vi "Build.vi"(6 "Version":T2, 7 "Build Events":refnum<class "Build Events API.lvclass">, 8 "error in (no error)":errorcluster, 10 "Build Info":T1, 11 "App Build in":refnum<class "App Build.lvclass">) -> (0 "error out":errorcluster)   [LabVIEW 2020, in "Builder Tools.lvlib" / "App Build.lvclass"]
uses:
  App Build.lvclass
  Builder Core/Version.ctl
  Build Events API/Build Events API.lvclass
  Build Info.ctl
  App Build.lvclass/App Build.ctl
  <vilib>/AppBuilder/AB_API_Simple/NI_App_Builder_API.lvlib
  <vilib>/AppBuilder/AB_API/Build/NI_AB_API_Build.lvclass
  <vilib>/AppBuilder/AB_API/common/AB_API Build Object Selector.ctl
  Builder Tools.lvlib
  <vilib>/AppBuilder/AB_API_Simple/Set Build Specification Version (path).vi
  Builder Core/Builder Core.lvlib
panel:
  out "Progress":i32
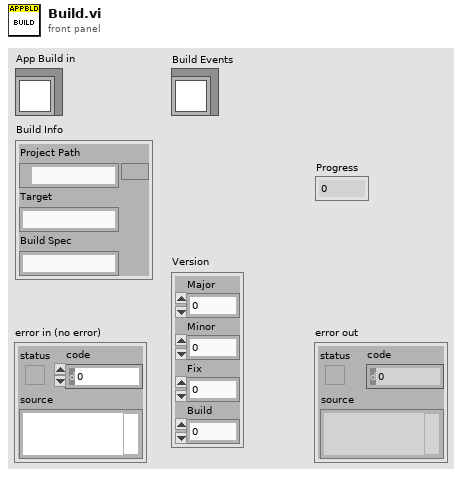
[diagram p1: front panel]
types:
  T1 = typedef "Builder Tools.lvlib/Build Info.ctl" = cluster{"Project Path":path, "Target":string, "Build Spec":string}
  T2 = typedef "Builder Core.lvlib/Version.ctl" = cluster{"Major":u16, "Minor":u16, "Fix":u16, "Build":u16}
  T3 = typedef "AB_API Build Object Selector.ctl" = enum16{"Source Distribution", "Deployable Source Distribution", "DLL", "EXE", "Packed Library", "Deployable Packed Library", "RT EXE", ".NET Interop Assembly"}
  T4 = typedef "AB_API ProgressBar_Events.ctl" = cluster{"newJob":refnum<user-event>, "newItem":refnum<user-event>, "errorMsg":T5, "cancel":refnum<user-event>}
  T5 = typedef "AB_API ProgressBar_BuildError.ctl" = refnum<user-event>
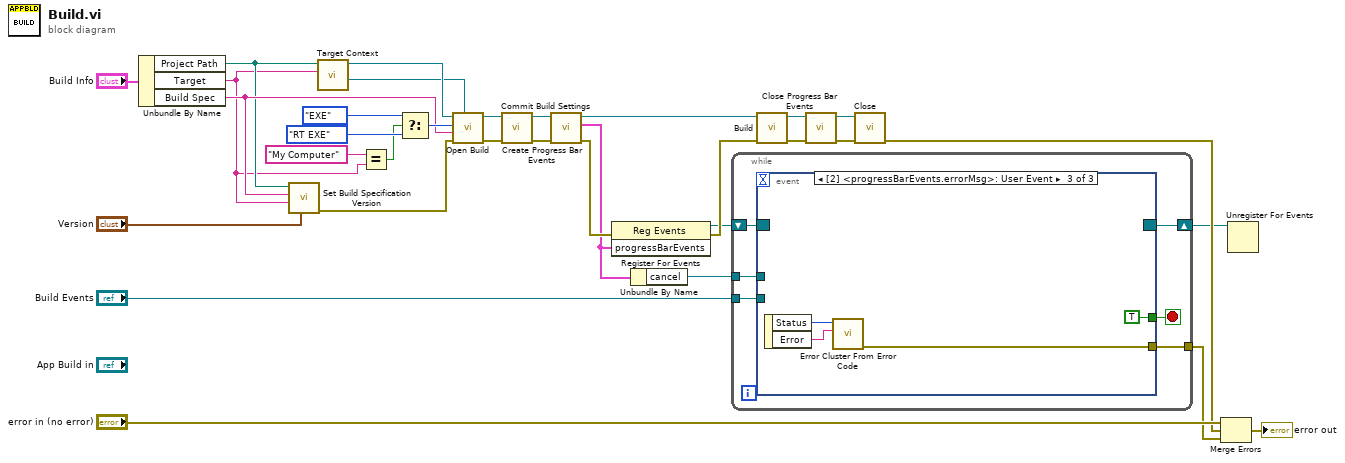
[diagram p0: block diagram]
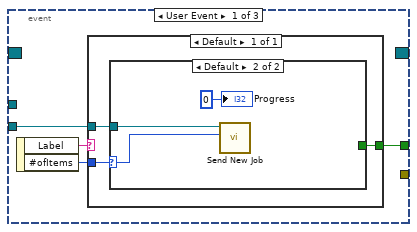
[diagram p2: hidden frame]
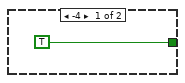
[diagram p3: hidden frame]
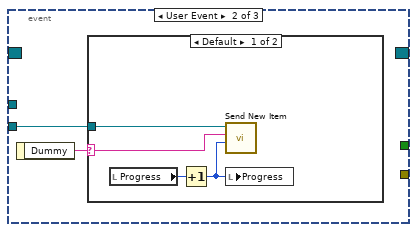
[diagram p4: hidden frame]
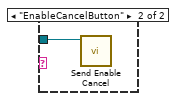
[diagram p5: hidden frame]
diagram:
  n1 = Unbundle By Name("Build Info") -> ("Project Path"=w22:path, "Target"=w21:string, "Build Spec"=w23:string)
  n2 = call-poly <vilib>:"Set Build Specification Version.vi"("Build Specification Version"="Version", "Name of target (My Computer)"=w21, "Name of build specification"=w23, "Path to project"=w22) -> ("error out"=w24:errorcluster)  [unwired: 7 in]
  n3 = call "Target Context.vi"("Target Name"=w21, "Project Path"=w22) -> ("Target"=w19:refnum<vi>, "Project"=w20:refnum<vi>)  [unwired: 7 in, 1 out]
  n4 = Equal?(x="My Computer", y=w21) -> (x = y?=w26:bool)
  n5 = Select(t=AB_API_Build_Object_Selector."EXE" ("Build object selector"), s=w26, f=AB_API_Build_Object_Selector."RT EXE" ("Build object selector")) -> (s? t:f=w25:T3)
  n6 = call <vilib>:"Open Build.vi"("TargetItem Refnum"=w19, "error in (no error)"=w24, "Build specification name"=w23, "Build object selector"=w25, "Project Refnum"=w20) -> ("error out"=w18:errorcluster, "NI_AB_API_Build out"=w17:refnum<class "NI_AB_API_Build.lvclass">)  [unwired: 5 in]
  n7 = call-dynamic "Commit Build Settings.vi"("error in (no error)"=w18, "Build in"=w17) -> ("error out"=w15:errorcluster, "Build out"=w16:refnum<class "NI_AB_API_Build.lvclass">)  [unwired: 8 in]
  n8 = call-dynamic "Create Progress Bar Events.vi"("error in (no error)"=w15, "NI_AB_API_Build in"=w16) -> ("error out"=w14:errorcluster, "progressBarEvents"=w13:T4, "NI_AB_API_Build out"=w10:refnum<class "NI_AB_API_Build.lvclass">)  [unwired: 7 in]
  n9 = register-events(error in=w14, w13) -> (reference out=w12:refnum<event-registration>, error out=w33:errorcluster)  [unwired: 1 in]
  n10 = Unbundle By Name(w13) -> ("cancel"=w11:refnum<user-event>)
  n11 = while {
    shift-right: [w36] -> w3
    shift-left: w12 -> [w39]
    tunnel: w11 -> [w38]
    tunnel: "Build Events" -> [w37]
    tunnel: [w34] -> w1
    stop <- w35 stop-if-true
    n12 = event shown="[2] <progressBarEvents.errorMsg>: User Event" {
      selector: w39 -> [_ _ _]
      dyn-events: [_ _ _] -> w36
      timeout: _ -> [_ _ _]
      tunnel: w38 -> [_ _ _]
      tunnel: w37 -> [w43 w51 _]
      tunnel: [w40 _ TRUE] -> w35
      tunnel: [_ _ w58] -> w34
      event User Event {
        n13 = event-data() -> ("Label"=w42:string, "#ofItems"=w41:i32)  [unwired: 1 in]
        n14 = case shown="Default" w42 {
          tunnel: w43 -> [w46]
          tunnel: w41 -> [w45]
          tunnel: [w44] -> w40
          frame Default {
            n15 = case shown="Default" w45 {
              selector: w45 -> [_ w49]
              tunnel: w46 -> [_ w50]
              tunnel: [TRUE _] -> w44
              frame -4 {
              }
              frame Default {
                n16 = call "Send New Job.vi"("Max Progress"=w49, "Build Events API in"=w50) -> ()  [unwired: 8 in, 2 out]
                "Progress" <- 0 ("Progress")
              }
            }
          }
        }
      }
      event User Event {
        n17 = event-data() -> ("Dummy"=w52:string)  [unwired: 1 in]
        n18 = case shown="Default" w52 {
          selector: w52 -> [w53 _]
          tunnel: w51 -> [w56 w57]
          frame Default {
            n19 = local read "Progress"() -> (w55:i32)
            n20 = Increment(x=w55) -> (x+1=w54:i32)
            n21 = call "Send New Item.vi"("Progress (0)"=w54, "Message"=w53, "Build Events API in"=w56) -> ()  [unwired: 7 in, 2 out]
            n22 = local write "Progress"(w54) -> ()
          }
          frame "EnableCancelButton" {
            n23 = call "Send Enable Cancel.vi"("Build Events API in"=w57) -> ()  [unwired: 9 in, 2 out]
          }
        }
      }
      event User Event {
        n24 = event-data() -> ("Status"=w61:i32, "Error"=w60:string)  [unwired: 1 in]
        n25 = call <vilib>:"Error Cluster From Error Code.vi"("error message (\"\")"=w60, "error code (0)"=w61) -> ("error out"=w58:errorcluster)  [unwired: 7 in]
      }
    }
  }
  n26 = call-dynamic "Build.vi"("error in (no error)"=w33, "Build in"=w10) -> ("error out"=w9:errorcluster, "Build out"=w8:refnum<class "NI_AB_API_Build.lvclass">)  [unwired: 6 in, 2 out]
  n27 = call-dynamic "Close Progress Bar Events.vi"("error in (no error)"=w9, "NI_AB_API_Build in"=w8) -> ("error out"=w7:errorcluster, "NI_AB_API_Build out"=w6:refnum<class "NI_AB_API_Build.lvclass">)  [unwired: 8 in]
  n28 = call-dynamic "Close.vi"("error in (no error)"=w7, "NI_AB_API_Build in"=w6) -> ("error out"=w4:errorcluster)  [unwired: 9 in]
  n29 = Merge Errors("error in (no error)", w4, w1) -> (→"error out":errorcluster)
  n30 = Unregister For Events(event registration refnum=w3) -> ()  [unwired: 1 in, 1 out]
